vi "File Dialog.vi"(8 "error in (no error)":errorcluster, 10 "Overwrite?":bool, 11 "Path In":path) -> (0 "error out":errorcluster, 3 "Path Out":path)   [LabVIEW 2019]
doc: "File Dialog\n\n<b>Development System</b>\n\nIf the path is not valid, this VI displays a File dialog box to choose the name of a new file.\n\n<b>Run Time System</b>\n\nNo dialog box.\nNo verification for file writes permission.\nIf the directory is not valid: \"Default Data Directory\" + \"PDF Report\" directory (Default Data Directory/ PDF Report).\n\n\n\nVersion 1.1\nDeveloped by Jean-Marc Simard\nCopyright © 2010, Exaprom Inc.\nAll rights reserved.\nLicense: BSD"
uses:
  <userlib>/Exaprom PDF/VIs/Low level/General/Stop if it True.vi
  <userlib>/Exaprom PDF/VIs/Low level/General/Continue if it True.vi
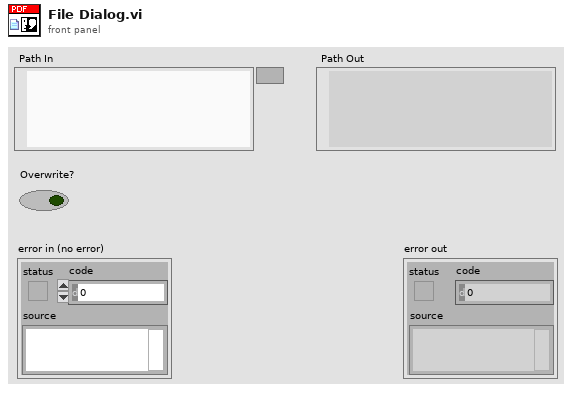
[diagram p1: front panel]
types:
  T1 = enum32{"invalid app kind", "Development System", "Run Time System", "Student Edition", "Embedded LabVIEW", "Evaluation", "Custom"}
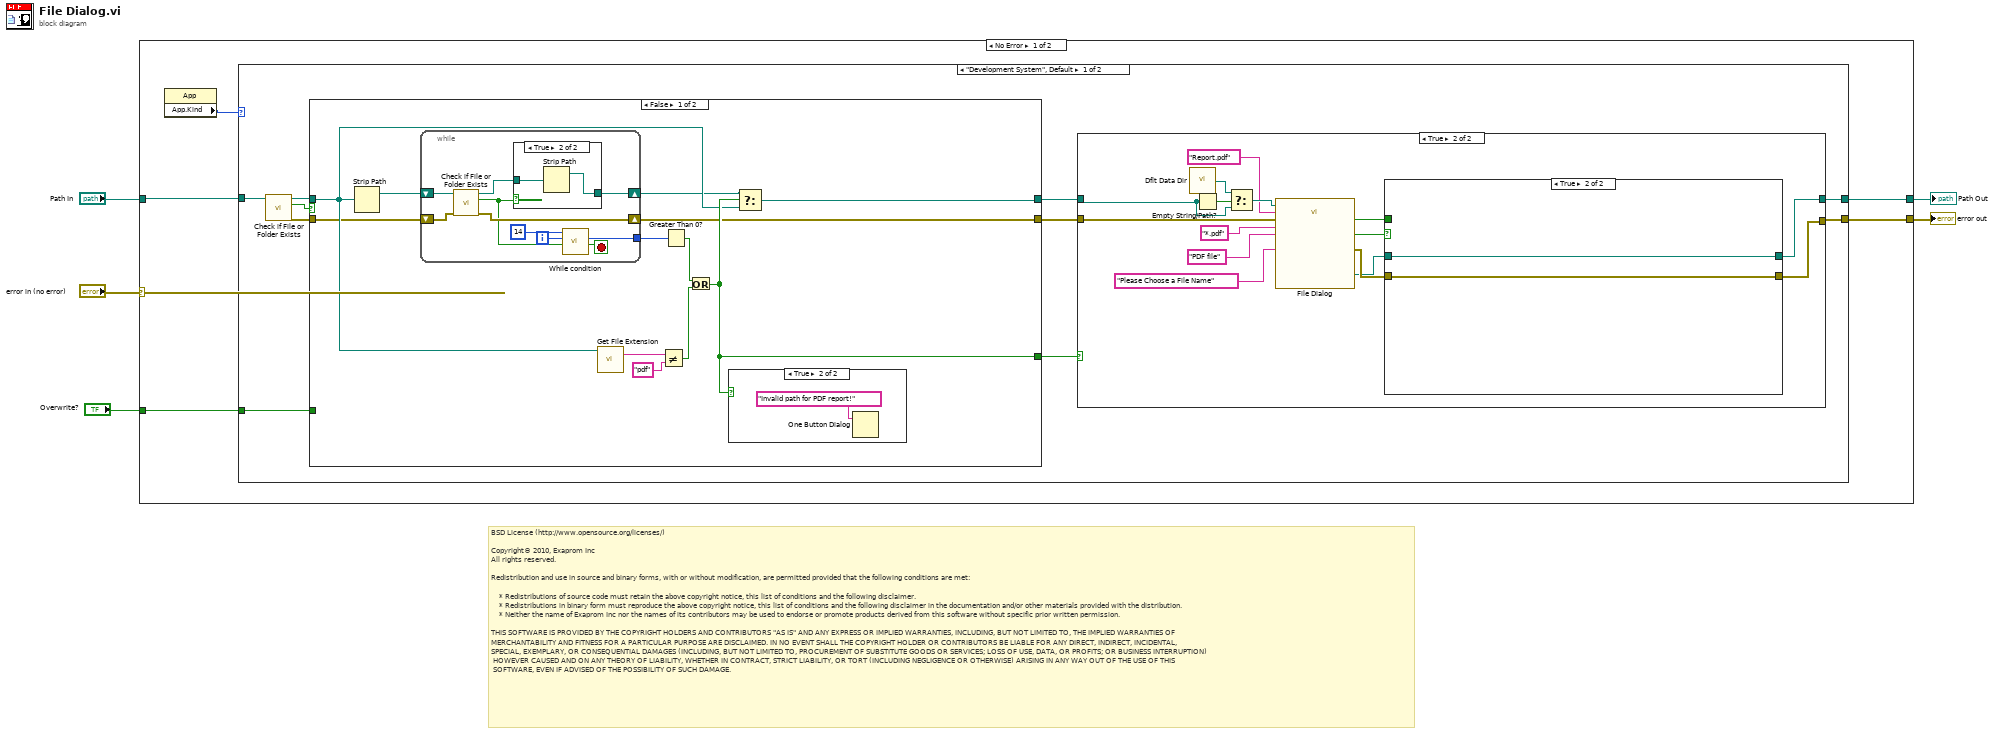
[diagram p0: block diagram]
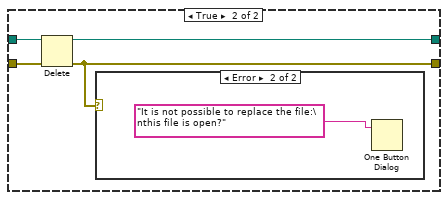
[diagram p4: hidden frame]
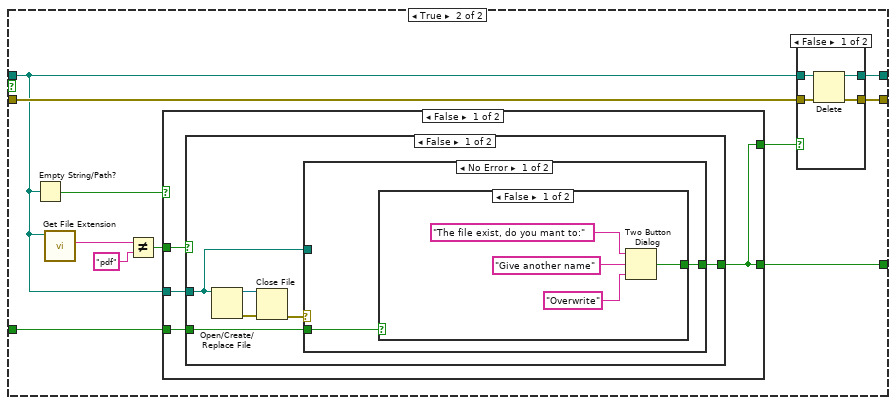
[diagram p8: hidden frame]
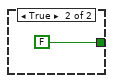
[diagram p9: hidden frame]
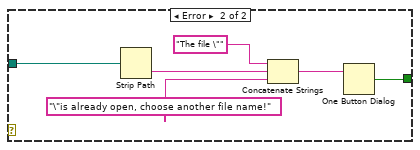
[diagram p10: hidden frame]
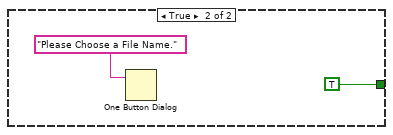
[diagram p11: hidden frame]
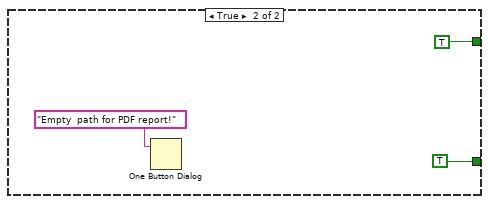
[diagram p12: hidden frame]
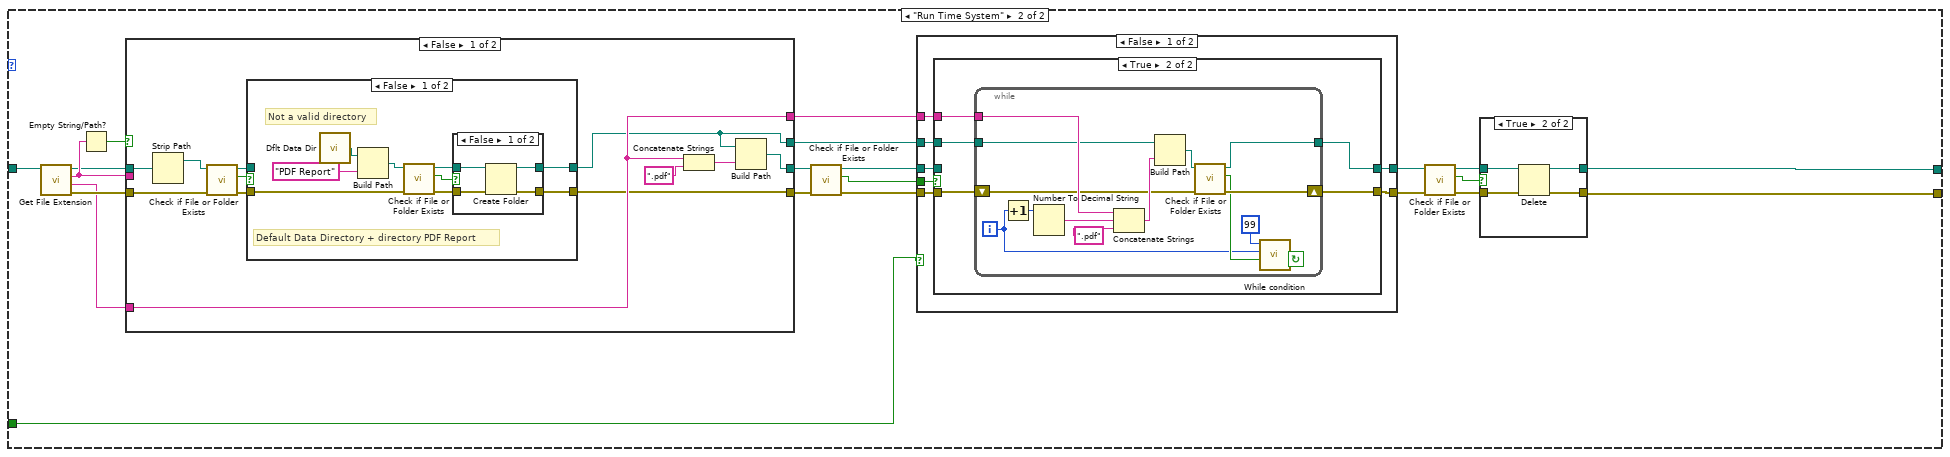
[diagram p14: hidden frame]
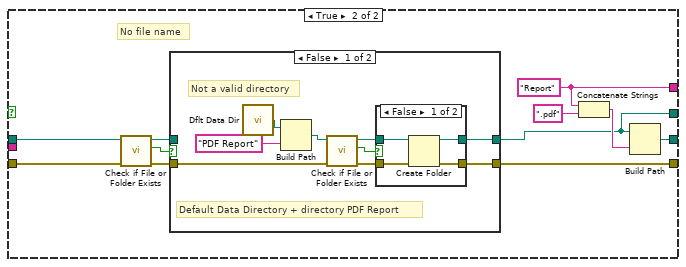
[diagram p20: hidden frame]
diagram:
  # "BSD License (http://www.opensource.org/licenses/)\n\nCopyright© 2010, Exaprom Inc\nAll rights reserved.\n\nRedistribution and use in source and binary forms, with or without modification, are permitted provided that the following conditions are met:\n\n    * Redistributions of source code must retain the above copyright notice, this list of conditions and the following disclaimer.\n    * Redistributions in binary form must reproduce the above copyright notice, this list of conditions and the following disclaimer in the documentation and/or other materials provided with the distribution.\n    * Neither the name of Exaprom Inc nor the names of its contributors may be used to endorse or promote products derived from this software without specific prior written permission.\n\nTHIS SOFTWARE IS PROVIDED BY THE COPYRIGHT HOLDERS AND CONTRIBUTORS \"AS IS\" AND ANY EXPRESS OR IMPLIED WARRANTIES, INCLUDING, BUT NOT LIMITED TO, THE IMPLIED WARRANTIES OF \nMERCHANTABILITY AND FITNESS FOR A PARTICULAR PURPOSE ARE DISCLAIMED. IN NO EVENT SHALL THE COPYRIGHT HOLDER OR CONTRIBUTORS BE LIABLE FOR ANY DIRECT, INDIRECT, INCIDENTAL,\nSPECIAL, EXEMPLARY, OR CONSEQUENTIAL DAMAGES (INCLUDING, BUT NOT LIMITED TO, PROCUREMENT OF SUBSTITUTE GOODS OR SERVICES; LOSS OF USE, DATA, OR PROFITS; OR BUSINESS INTERRUPTION)\n HOWEVER CAUSED AND ON ANY THEORY OF LIABILITY, WHETHER IN CONTRACT, STRICT LIABILITY, OR TORT (INCLUDING NEGLIGENCE OR OTHERWISE) ARISING IN ANY WAY OUT OF THE USE OF THIS\n SOFTWARE, EVEN IF ADVISED OF THE POSSIBILITY OF SUCH DAMAGE."
  n1 = case shown="No Error" "error in (no error)" {
    selector: "error in (no error)" -> [_ w238]
    tunnel: [w9 w238] -> w5
    tunnel: "Path In" -> [w6 w237]
    tunnel: [w10 w237] -> w2
    tunnel: "Overwrite?" -> [w8 _]
    frame No Error {
      n2 = property class="App"() -> ("App.Kind"=w7:T1)  [unwired: 2 in, 2 out]
      n3 = case shown="\"Development System\", Default" w7 {
        tunnel: [w17 w124] -> w10
        tunnel: [w16 w123] -> w9
        tunnel: w6 -> [w14 w132]
        tunnel: w8 -> [w15 w130]
        frame "Development System", Default {
          n4 = call <vilib>:"Check if File or Folder Exists.vi"("path"=w14) -> ("error out"=w11:errorcluster, "file or folder exists?"=w12:bool, "dup path"=w13:path)  [unwired: 1 in, 7 out]
          n5 = case shown="False" w12 {
            tunnel: w13 -> [w58 w80]
            tunnel: [w59 w88] -> w19
            tunnel: w11 -> [w54 w86]
            tunnel: [w55 w87] -> w18
            tunnel: [w60 w85] -> w20
            tunnel: w15 -> [_ w78]
            frame False {
              n6 = Strip Path(path=w58) -> (stripped path=w53:path)  [unwired: 1 out]
              n7 = while {
                shift-right: [w71] -> w56
                shift-left: w53 -> [w73]
                shift-right: [w70] -> w55
                shift-left: w54 -> [w69]
                tunnel: [w66] -> w52
                i -> [w65]
                stop <- w67 stop-if-true
                n8 = call <vilib>:"Check if File or Folder Exists.vi"("error in (no error)"=w69, "path"=w73) -> ("error out"=w70:errorcluster, "file or folder exists?"=w68:bool, "dup path"=w72:path)  [unwired: 7 out]
                n9 = case shown="True" w68 {
                  tunnel: w72 -> [w74 w76]
                  tunnel: [w74 w75] -> w71
                  frame False {
                  }
                  frame True {
                    n10 = Strip Path(path=w76) -> (stripped path=w75:path)  [unwired: 1 out]
                  }
                }
                n11 = call-poly <userlib>:"While condition.vi"("Test"=w68, "i"=w65, "N"=14) -> ("Action"=w67:bool, "i duplicate"=w66:i32)  [unwired: 4 out]
              }
              n12 = call <vilib>:"Get File Extension.vi"("file"=w58) -> ("lowercase file extension"=w57:string)  [unwired: 1 in, 9 out]
              n13 = Not Equal?(x=w57, y="pdf") -> (x != y?=w62:bool)
              n14 = Greater Than 0?(x=w52) -> (x > 0?=w61:bool)
              n15 = Or(x=w61, y=w62) -> (x .or. y?=w60:bool)
              n16 = case shown="True" w60 {
                frame False {
                }
                frame True {
                  n17 = One Button Dialog(message="Invalid path for PDF report!") -> ()  [unwired: 2 out]
                }
              }
              n18 = Select(t=w56, s=w60, f=w58) -> (s? t:f=w59:path)
            }
            frame True {
              n19 = Empty String/Path?(string/path=w80) -> (empty?=w84:bool)
              n20 = call <vilib>:"Get File Extension.vi"("file"=w80) -> ("lowercase file extension"=w79:string)  [unwired: 1 in, 9 out]
              n21 = Not Equal?(x=w79, y="pdf") -> (x != y?=w81:bool)
              n22 = case shown="False" w84 {
                tunnel: [w92 TRUE ("T button?")] -> w85
                tunnel: [w92 TRUE] -> w83
                tunnel: w81 -> [w91 _]
                tunnel: w80 -> [w90 _]
                tunnel: w78 -> [w89 _]
                frame False {
                  n23 = case shown="False" w91 {
                    tunnel: [w98 TRUE] -> w92
                    tunnel: w90 -> [w94 _]
                    tunnel: w89 -> [w93 _]
                    frame False {
                      n24 = Open/Create/Replace File(file path (use dialog)=w94) -> (refnum out=w96:refnum<file>, error out=w97:errorcluster)  [unwired: 1 in, 5 out]
                      n25 = Close File(refnum=w96, error in=w97) -> (error out=w95:errorcluster)  [unwired: 1 out]
                      n26 = case shown="No Error" w95 {
                        tunnel: [w100 w111] -> w98
                        tunnel: w94 -> [_ w106]
                        tunnel: w93 -> [w99 _]
                        frame No Error {
                          n27 = case shown="False" w99 {
                            tunnel: [w101 FALSE] -> w100
                            frame False {
                              n28 = Two Button Dialog(message="The file exist, do you mant to:", 1:"Overwrite" ("T button name (\"OK\")"), 2:"Give another name" ("F button name (\"Cancel\")")) -> (T button?=w101:bool)
                            }
                            frame True {
                            }
                          }
                        }
                        frame Error {
                          n29 = Strip Path(path=w106) -> (name=w109:string)  [unwired: 1 out]
                          n30 = Concatenate Strings("The file \"", w109, "\"is already open, choose another file name!") -> (w107:string)
                          n31 = One Button Dialog(message=w107) -> (true=w111:bool)  [unwired: 1 out]
                        }
                      }
                    }
                    frame True {
                      n32 = One Button Dialog(message="Please Choose a File Name." ("prompt")) -> ()  [unwired: 2 out]
                    }
                  }
                }
                frame True {
                  n33 = One Button Dialog(message="Empty  path for PDF report!") -> ()  [unwired: 2 out]
                }
              }
              n34 = case shown="False" w83 {
                tunnel: [w120 w122] -> w88
                tunnel: [w119 w121] -> w87
                tunnel: w86 -> [w118 w121]
                tunnel: w80 -> [w117 w122]
                frame False {
                  n35 = Delete(path (use dialog)=w117, error in=w118) -> (deleted path=w120:path, error out=w119:errorcluster)  [unwired: 4 out]
                }
                frame True {
                }
              }
            }
          }
          n36 = case shown="True" w20 {
            tunnel: w19 -> [w22 w33]
            tunnel: [w22 w25] -> w17
            tunnel: w18 -> [w21 w36]
            tunnel: [w21 w26] -> w16
            frame False {
            }
            frame True {
              n37 = call <vilib>:"Dflt Data Dir.vi"() -> ("App:Default Data Directory"=w24:path)
              n38 = Empty String/Path?(string/path=w33) -> (empty?=w34:bool)
              n39 = Select(t=w24, s=w34, f=w33) -> (s? t:f=w32:path)
              n40 = call "File Dialog"("start path"=w32, "prompt"="Please Choose a File Name", "default name"="Report.pdf", "error in"=w36, "pattern (all files)"="*.pdf", "pattern label"="PDF file") -> ("selected path"=w27:path, "exists"=w29:bool, "cancelled"=w30:bool, "error out"=w28:errorcluster)  [unwired: 1 in, 5 out]
              n41 = case shown="True" w30 {
                tunnel: w29 -> [w42 _]
                tunnel: w28 -> [w41 w51]
                tunnel: w27 -> [w40 w50]
                tunnel: [w39 w51] -> w26
                tunnel: [w38 w50] -> w25
                frame False {
                  n42 = case shown="False" w42 {
                    tunnel: w41 -> [w43 w48]
                    tunnel: w40 -> [w44 w47]
                    tunnel: [w43 w45] -> w39
                    tunnel: [w44 w46] -> w38
                    frame False {
                    }
                    frame True {
                      n43 = Delete(path (use dialog)=w47, error in=w48) -> (deleted path=w46:path, error out=w45:errorcluster)  [unwired: 4 out]
                      n44 = case shown="Error" w45 {
                        frame No Error {
                        }
                        frame Error {
                          n45 = One Button Dialog(message="It is not possible to replace the file:\nthis file is open?" ("prompt")) -> ()  [unwired: 2 out]
                        }
                      }
                    }
                  }
                }
                frame True {
                }
              }
            }
          }
        }
        frame "Run Time System" {
          n46 = call <vilib>:"Get File Extension.vi"("file"=w132) -> ("error out"=w134:errorcluster, "filename without extension"=w133:string, "lowercase file extension"=w137:string, "dup file"=w135:path)  [unwired: 1 in, 6 out]
          n47 = Empty String/Path?(string/path=w137) -> (empty?=w136:bool)
          n48 = case shown="False" w136 {
            tunnel: w137 -> [_ _]
            tunnel: w135 -> [w187 w219]
            tunnel: w134 -> [w183 w218]
            tunnel: [w191 w213] -> w139
            tunnel: [w182 w215] -> w138
            tunnel: w133 -> [w188 _]
            tunnel: [w188 w210] -> w141
            tunnel: [w180 w209] -> w140
            frame False {
              n49 = Strip Path(path=w187) -> (stripped path=w181:path)  [unwired: 1 out]
              n50 = call <vilib>:"Check if File or Folder Exists.vi"("error in (no error)"=w183, "path"=w181) -> ("error out"=w184:errorcluster, "file or folder exists?"=w185:bool, "dup path"=w186:path)  [unwired: 7 out]
              n51 = case shown="False" w185 {
                tunnel: w184 -> [w197 w207]
                tunnel: [w193 w208] -> w180
                tunnel: [w192 w207] -> w182
                tunnel: w186 -> [_ w208]
                frame False {
                  # "Not a valid directory"
                  # "Default Data Directory + directory PDF Report"
                  n52 = call <vilib>:"Dflt Data Dir.vi"() -> ("App:Default Data Directory"=w200:path)
                  n53 = Build Path(base path=w200, name or relative path="PDF Report") -> (appended path=w198:path)
                  n54 = call <vilib>:"Check if File or Folder Exists.vi"("error in (no error)"=w197, "path"=w198) -> ("error out"=w195:errorcluster, "file or folder exists?"=w196:bool, "dup path"=w194:path)  [unwired: 7 out]
                  n55 = case shown="False" w196 {
                    tunnel: w195 -> [w204 w205]
                    tunnel: w194 -> [w203 w206]
                    tunnel: [w202 w206] -> w193
                    tunnel: [w201 w205] -> w192
                    frame False {
                      n56 = Create Folder(path (use dialog)=w203, error in=w204) -> (created path=w202:path, error out=w201:errorcluster)  [unwired: 2 out]
                    }
                    frame True {
                    }
                  }
                }
                frame True {
                }
              }
              n57 = Concatenate Strings(w188, ".pdf" ("y")) -> (w189:string)
              n58 = Build Path(base path=w180, name or relative path=w189) -> (appended path=w191:path)
            }
            frame True {
              w210 = "Report" ("filename without extension")
              # "No file name"
              n59 = call <vilib>:"Check if File or Folder Exists.vi"("error in (no error)"=w218, "path"=w219) -> ("error out"=w216:errorcluster, "file or folder exists?"=w217:bool, "dup path"=w214:path)  [unwired: 7 out]
              n60 = case shown="False" w217 {
                tunnel: w216 -> [w225 w235]
                tunnel: [w221 w236] -> w209
                tunnel: [w220 w235] -> w215
                tunnel: w214 -> [_ w236]
                frame False {
                  # "Not a valid directory"
                  # "Default Data Directory + directory PDF Report"
                  n61 = call <vilib>:"Dflt Data Dir.vi"() -> ("App:Default Data Directory"=w228:path)
                  n62 = Build Path(base path=w228, name or relative path="PDF Report") -> (appended path=w226:path)
                  n63 = call <vilib>:"Check if File or Folder Exists.vi"("error in (no error)"=w225, "path"=w226) -> ("error out"=w223:errorcluster, "file or folder exists?"=w224:bool, "dup path"=w222:path)  [unwired: 7 out]
                  n64 = case shown="False" w224 {
                    tunnel: w223 -> [w232 w233]
                    tunnel: w222 -> [w231 w234]
                    tunnel: [w230 w234] -> w221
                    tunnel: [w229 w233] -> w220
                    frame False {
                      n65 = Create Folder(path (use dialog)=w231, error in=w232) -> (created path=w230:path, error out=w229:errorcluster)  [unwired: 2 out]
                    }
                    frame True {
                    }
                  }
                }
                frame True {
                }
              }
              n66 = Concatenate Strings(w210, ".pdf" ("y")) -> (w211:string)
              n67 = Build Path(base path=w209, name or relative path=w211) -> (appended path=w213:path)
            }
          }
          n68 = call <vilib>:"Check if File or Folder Exists.vi"("error in (no error)"=w138, "path"=w139) -> ("error out"=w142:errorcluster, "file or folder exists?"=w131:bool, "dup path"=w143:path)  [unwired: 7 out]
          n69 = case shown="False" w130 {
            tunnel: w143 -> [w156 w178]
            tunnel: w142 -> [w155 w179]
            tunnel: w141 -> [w154 _]
            tunnel: w140 -> [w153 _]
            tunnel: [w152 w178] -> w128
            tunnel: [w151 w179] -> w129
            tunnel: w131 -> [w150 _]
            frame False {
              n70 = case shown="True" w150 {
                tunnel: w153 -> [_ w162]
                tunnel: w154 -> [_ w163]
                tunnel: w155 -> [w158 w161]
                tunnel: [w157 w159] -> w152
                tunnel: [w158 w160] -> w151
                tunnel: w156 -> [w157 _]
                frame False {
                }
                frame True {
                  n71 = while {
                    tunnel: w163 -> [w176]
                    shift-right: [w170] -> w160
                    shift-left: w161 -> [w172]
                    tunnel: w162 -> [w169]
                    tunnel: [w168] -> w159
                    i -> [w165]
                    stop <- w167 continue-if-true
                    n72 = Increment(x=w165) -> (x+1=w177:i32)
                    n73 = Number To Decimal String(number=w177) -> (decimal integer string=w175:string)  [unwired: 1 out]
                    n74 = Concatenate Strings(w176, w175, ".pdf" ("y")) -> (w173:string)
                    n75 = Build Path(base path=w169, name or relative path=w173) -> (appended path=w171:path)
                    n76 = call <vilib>:"Check if File or Folder Exists.vi"("error in (no error)"=w172, "path"=w171) -> ("error out"=w170:errorcluster, "file or folder exists?"=w166:bool, "dup path"=w168:path)  [unwired: 7 out]
                    n77 = call-poly <userlib>:"While condition.vi"("Test"=w166, "i"=w165, "N"=99) -> ("Action"=w167:bool)  [unwired: 5 out]
                  }
                }
              }
            }
            frame True {
            }
          }
          n78 = call <vilib>:"Check if File or Folder Exists.vi"("error in (no error)"=w129, "path"=w128) -> ("error out"=w126:errorcluster, "file or folder exists?"=w125:bool, "dup path"=w127:path)  [unwired: 7 out]
          n79 = case shown="True" w125 {
            tunnel: w126 -> [w144 w149]
            tunnel: [w144 w147] -> w123
            tunnel: w127 -> [w145 w148]
            tunnel: [w145 w146] -> w124
            frame False {
            }
            frame True {
              n80 = Delete(path (use dialog)=w148, error in=w149) -> (deleted path=w146:path, error out=w147:errorcluster)  [unwired: 4 out]
            }
          }
        }
      }
    }
    frame Error {
    }
  }
  "error out" <- w5
  "Path Out" <- w2
